vi "Authorization Get Auth.vi"(8 "error in (no error)":errorcluster, 11 "Debug?":bool) -> (0 "error out":errorcluster, 3 "Authorization":T1)   [LabVIEW 2011]
doc: "GetAuthorization() gets the level at which the protected program is authorized to run along with the options enabled or an authorization failure code. It is also used to decrement the number of runs, if the application is restricted by runs.\n\nGetAuthorization() can be called at your discretion to determine the level of authorization that the user is granted. It can also be called to decrement the number of uses the program has left if it is restricted by number of runs. Call this function after calling any function that changes the license state, such as SaveSiteKey(), TransferOut() or TransferIn(), so that the program can alter its behavior according to the change that has occurred.\n\nValue Meaning\n>0 The program is authorized to run. The program has a floating license and more users are requesting to use the program than the license allows. The number indicates how many users must quit before the next user is authorized to run. CrypKey queues requests for access and provides access on a first-come, first-served basis.\n0 The program is authorized to run.\n-1 CrypKey has not been initialized.\n-2 An attempt is being made to run the protected program from a floppy disk.\n-3 Could not read the site key file.\n-4 The program has never been authorized at the current site.\n-5 The program is moved or the password is incorrect.\n-6 The Master Key is not correct for this program.\n-7 The site key file is damaged or tampered with.\n-8 The system time is set to a date earlier than the date on which the Site Key was issued.\n-9 The program is restricted by days and the system time is set back.\n-10 The program is restricted by days and the time has expired.\n-11 The program is restricted by runs and the number allowed is reached.\n-12 The user tried to perform an operation that requires more runs than are available.\n-13 The restriction file is deleted.\n-14 The restriction file is damaged or tampered with.\n-15 The restriction file is moved or overwritten.\n-16 The user has attempted to reuse an old site key.\n-17 Could not open or read the network user table file.\n-18 More people are using the protected program than SLAPI can handle.\n-19 An attempt is being made to run the program in client/server mode and a floating license has not been issued for the site.\n-20 .RST file is write protected \n-21 Computer clock tampering detected \n-22 Application site key is moved or copied \n\nThe options are single bits of information that can be turned on or off individually when a license is created using the Site Key Generator. The options exist so that you can turn on or off different features of your product. The options are stored in a numerical sequence starting at one with the high-end bit of the oplevel 32-bit value. The remaining bits are used to hold the level number.\nThe level is a number that is set by the Site Key Generator. It incrementally controls the quality of some services your software provides, such as the number of records allowed for a database. The maximum level depends on the number of options you have configured.\nThere are 32 bits available to both the option and level values."
uses:
  Authorization Data.ctl
  Authorization Global.vi
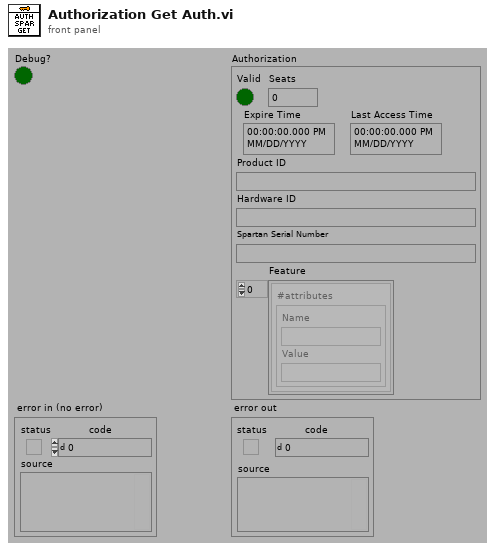
[diagram p1: front panel]
types:
  T1 = typedef "Authorization Data.ctl" = cluster{"Valid":bool, "Seats":i32, "Expire Time":timestamp, "Last Access Time":timestamp, "Product ID":string, "Hardware ID":string, "Spartan Serial Number":string, "Feature":cluster{"#attributes":cluster{"Name":string, "Value":string}}[]}
  T2 = enum32{"invalid app kind", "Development System", "Run Time System", "Student Edition", "Embedded LabVIEW", "Evaluation", "Custom"}
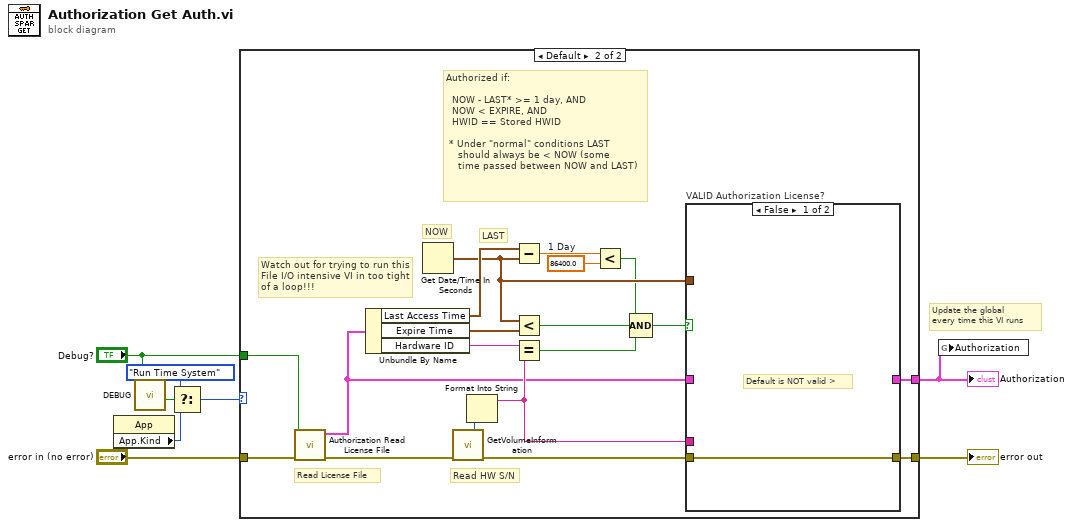
[diagram p0: block diagram]
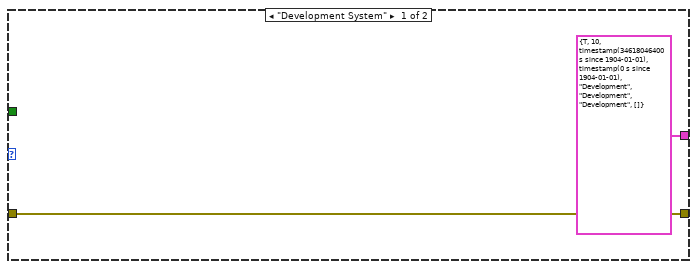
[diagram p2: hidden frame]
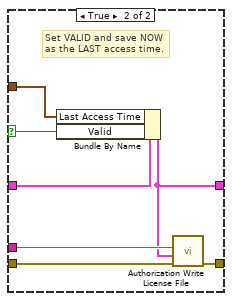
[diagram p3: hidden frame]
diagram:
  # "Update the global\nevery time this VI runs"
  n1 = property class="App"() -> ("App.Kind"=w3:T2)  [unwired: 2 in, 2 out]
  n2 = call "DEBUG.vi"("Dev DEBUG? (f)"="Debug?") -> ("DEBUG?"=w5:bool)  [unwired: 1 in, 5 out]
  n3 = Select(t=T2."Run Time System", s=w5, f=w3) -> (s? t:f=w2:T2)
  n4 = case shown="Default" w2 {
    tunnel: "error in (no error)" -> [w10 w29]
    tunnel: [w10 w28] -> w7
    tunnel: [T1 {"Valid"=TRUE, "Seats"=10, "Expire Time"=timestamp(34618046400 s since 1904-01-01), "Last Access Time"=timestamp(0 s since 1904-01-01), "Product ID"="Development", "Hardware ID"="Development", "Spartan Serial Number"="Development", "Feature"=[]} ("Authorization") w15] -> w6
    tunnel: "Debug?" -> [_ w11]
    frame "Development System" {
    }
    frame Default {
      w12 = 86400.0  # 1 Day
      # "Watch out for trying to run this\nFile I/O intensive VI in too tight\nof a loop!!!"
      # "LAST"
      # "Authorized if:\n\n  NOW - LAST* >= 1 day, AND\n  NOW < EXPIRE, AND\n  HWID == Stored HWID\n\n * Under \"normal\" conditions LAST\n    should always be < NOW (some\n    time passed between NOW and LAST)"
      # "NOW"
      # "Read HW S/N"
      # "Read License File"
      n5 = call "Authorization Read License File.vi"("error in (no error)"=w29, "Debug?"=w11) -> ("error out"=w22:errorcluster, "Authorization"=w16:T1)  [unwired: 8 in]
      n6 = Unbundle By Name(w16) -> ("Last Access Time"=w21:timestamp, "Expire Time"=w27:timestamp, "Hardware ID"=w25:string)
      n7 = Get Date/Time In Seconds() -> (seconds since 1Jan1904=w18:timestamp)
      n8 = call "GetVolumeInformation.vi"("error in (no error)"=w22) -> ("VolumeSerialNumber"=w26:u32, "error out"=w20:errorcluster)  [unwired: 8 in, 5 out]
      n9 = Format Into String(w26) -> (resulting string=w19:string)  [unwired: 3 in, 1 out]
      n10 = Subtract(x=w21, y=w18) -> (x-y=w13:dbl)
      n11 = Less?(x=w18, y=w27) -> (x < y?=w24:bool)
      n12 = Equal?(x=w25, y=w19) -> (x = y?=w23:bool)
      n13 = Less?(x=w13, y=w12) -> (x < y?=w17:bool)
      n14 = Compound Arithmetic op=AND(w17, w24, w23) -> (w14:bool)
      n15 = case "VALID Authorization License?" shown="False" w14 {
        selector: w14 -> [_ w31]
        tunnel: w20 -> [w30 w37]
        tunnel: [w30 w36] -> w28
        tunnel: w19 -> [_ w35]
        tunnel: w16 -> [_ w33]
        tunnel: w18 -> [_ w34]
        tunnel: [_ w32] -> w15
        frame False {
          # "Default is NOT valid >"
        }
        frame True {
          # "Set VALID and save NOW\nas the LAST access time."
          n16 = Bundle By Name(cluster=w33, "Last Access Time"=w34, "Valid"=w31) -> (w32:T1)
          n17 = call "Authorization Write License File.vi"("error in (no error)"=w37, "Authorization"=w32, "Hardware ID"=w35) -> ("error out"=w36:errorcluster)  [unwired: 8 in]
        }
      }
    }
  }
  "error out" <- w7
  "Authorization" <- w6
  n18 = global write "Authorization Global.vi" "Authorization"(w6) -> ()
